vi "Configure Trigger.vi"(0 "VISA resource name":refnum<visa-resource-name>, 1 "Trigger Type (0:Untriggered)":u16(ring) items=["Untriggered", "Software Triggered", "Hardware Triggered"], 5 "Trigger Start Edge (0: Rising)":u16(ring) items=["Rising", "Falling"], 7 "Trigger Stop Edge (0: Rising)":u16(ring) items=["Rising", "Falling"], 9 "Trigger Stop Condition (1:Edge Triggering)":u16(ring)=1 items=["Number of Acquisitions", "Edge Triggering"], 11 "error in (no error)":errorcluster, 12 "Number of Acquisitions (100)":i32=100, 13 "Enable Continuous Trigger (Disabled)":bool) -> (4 "VISA resource name out":refnum<visa-resource-name>, 6 "Response":string[](array[string]), 15 "error out":errorcluster)   [LabVIEW 2015, in "Micron Optics sm130.lvlib"]
doc: "Configures the trigger settings such as trigger type, start and stop edge, stop conditions, number of acquisitions and enable continuous trigger."
uses:
  Micron Optics sm130.lvlib
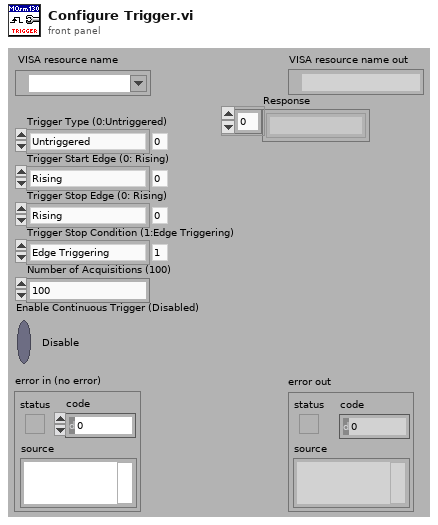
[diagram p1: front panel]
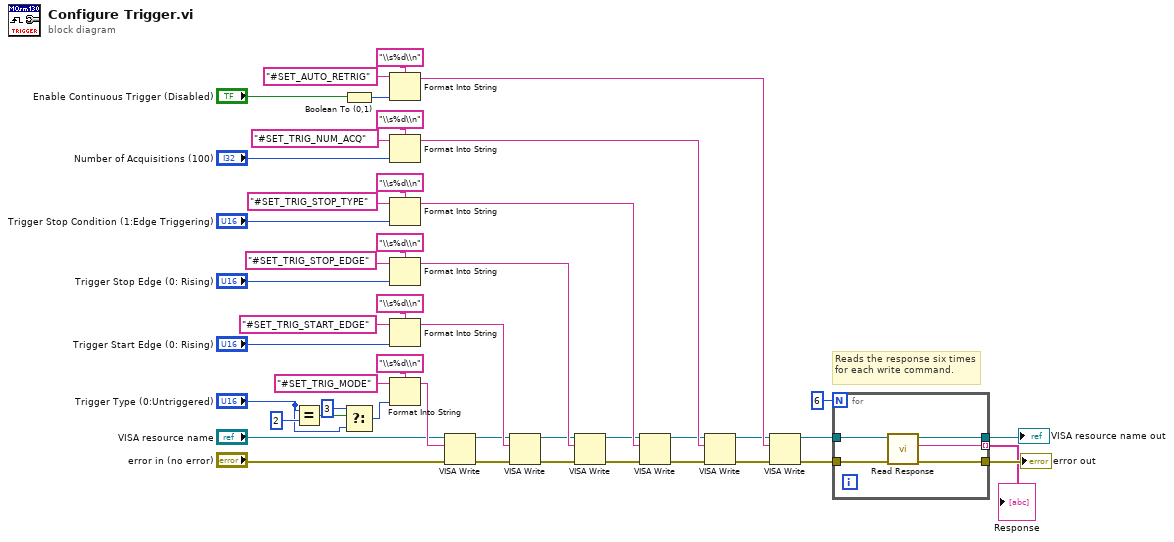
[diagram p0: block diagram]
diagram:
  # "Reads the response six times for each write command."
  n1 = Equal?(x="Trigger Type (0:Untriggered)", y=u16 2) -> (x = y?=w4:bool)
  n2 = Boolean To (0,1)(Boolean="Enable Continuous Trigger (Disabled)") -> (0, 1=w29:i16)
  n3 = Select(t=u16 3, s=w4, f="Trigger Type (0:Untriggered)") -> (s? t:f=w1:u16)
  n4 = Format Into String(format string="\\s%d\\n", initial string="#SET_AUTO_RETRIG", w29) -> (resulting string=w24:string)  [unwired: 1 in, 1 out]
  n5 = Format Into String(format string="\\s%d\\n", initial string="#SET_TRIG_NUM_ACQ", "Number of Acquisitions (100)") -> (resulting string=w25:string)  [unwired: 1 in, 1 out]
  n6 = Format Into String(format string="\\s%d\\n", initial string="#SET_TRIG_STOP_TYPE", "Trigger Stop Condition (1:Edge Triggering)") -> (resulting string=w26:string)  [unwired: 1 in, 1 out]
  n7 = Format Into String(format string="\\s%d\\n", initial string="#SET_TRIG_STOP_EDGE", "Trigger Stop Edge (0: Rising)") -> (resulting string=w27:string)  [unwired: 1 in, 1 out]
  n8 = Format Into String(format string="\\s%d\\n", initial string="#SET_TRIG_START_EDGE", "Trigger Start Edge (0: Rising)") -> (resulting string=w28:string)  [unwired: 1 in, 1 out]
  n9 = Format Into String(format string="\\s%d\\n", initial string="#SET_TRIG_MODE", w1) -> (resulting string=w45:string)  [unwired: 1 in, 1 out]
  n10 = VISA Write(VISA resource name="VISA resource name", write buffer=w45, error in (no error)="error in (no error)") -> (VISA resource name out=w12:refnum<visa-resource-name>, error out=w11:errorcluster)  [unwired: 1 out]
  n11 = VISA Write(VISA resource name=w12, write buffer=w28, error in (no error)=w11) -> (VISA resource name out=w14:refnum<visa-resource-name>, error out=w13:errorcluster)  [unwired: 1 out]
  n12 = VISA Write(VISA resource name=w14, write buffer=w27, error in (no error)=w13) -> (VISA resource name out=w15:refnum<visa-resource-name>, error out=w16:errorcluster)  [unwired: 1 out]
  n13 = VISA Write(VISA resource name=w15, write buffer=w26, error in (no error)=w16) -> (VISA resource name out=w18:refnum<visa-resource-name>, error out=w17:errorcluster)  [unwired: 1 out]
  n14 = VISA Write(VISA resource name=w18, write buffer=w25, error in (no error)=w17) -> (VISA resource name out=w20:refnum<visa-resource-name>, error out=w19:errorcluster)  [unwired: 1 out]
  n15 = VISA Write(VISA resource name=w20, write buffer=w24, error in (no error)=w19) -> (VISA resource name out=w22:refnum<visa-resource-name>, error out=w21:errorcluster)  [unwired: 1 out]
  n16 = for {
    N: 6 -> [_]
    tunnel: w22 -> [w52]
    tunnel: w21 -> [w51]
    tunnel: [w50] -> w8
    tunnel: [w49] -> w7
    tunnel: [w48] -> w6 mode=indexing
    n17 = call "Read Response.vi"("error in (no error)"=w51, "VISA resource name"=w52) -> ("error out"=w49:errorcluster, "Confirmation Response"=w48:string, "VISA resource name out"=w50:refnum<visa-resource-name>)  [unwired: 7 in]
  }
  "VISA resource name out" <- w8
  "error out" <- w7
  "Response" <- w6
